vi "4. Panel Control.vi"   [LabVIEW 2017, in "1. Basic Panels.lvlib"]
uses:
  1. Basic Panels.lvlib
  panel-manager/Source/MGI-Panel Manager.lvlib
  panel-manager/Source/Panel/Subpanel/Subpanel.vi
  panel-manager/Source/Panel/Subpanel/Subpanel.lvclass
  panel-manager/Source/Panel/Window/Window.vi
  panel-manager/Source/Panel/Window/Window.lvclass
  panel-manager/Source/Window Position/Reference Position/Ref Top Level/Ref Top Level.vi
  panel-manager/Source/Window Position/Reference Position/Ref Top Level/Ref Top Level.lvclass
  panel-manager/Source/Window Position/Reference Position/Size/Absolute Size/Min Panel Size.vi
  panel-manager/Source/Window Position/Reference Position/Size/Absolute Size/Absolute Size.lvclass
  panel-manager/Source/Window Position/Reference Position/Alignment.ctl
  panel-manager/Source/Window Position/Reference Position/Reference Position.lvclass
  panel-manager/Source/Window Position/Reference Position/Offset/Absolute Offset/Absolute Offset.lvclass
  panel-manager/Source/Window Position/Reference Position/Vertical Alignment.ctl
  panel-manager/Source/Window Position/Reference Position/Horizontal Alignment.ctl
  D:/software/LabView_PanelManager/panel-manager/Source/Panel/Panel.lvclass
  D:/software/LabView_PanelManager/panel-manager/Source/Window Position/Reference Position/Offset/Offset.lvclass
  D:/software/LabView_PanelManager/panel-manager/Source/Window Position/Reference Position/Size/Size.lvclass
  D:/software/LabView_PanelManager/panel-manager/Source/Window Position/Reference Position/Reference Position.lvclass
  D:/software/LabView_PanelManager/panel-manager/Source/Window Position/Window Position.lvclass
panel:
  # "Run this VI to view instructions"
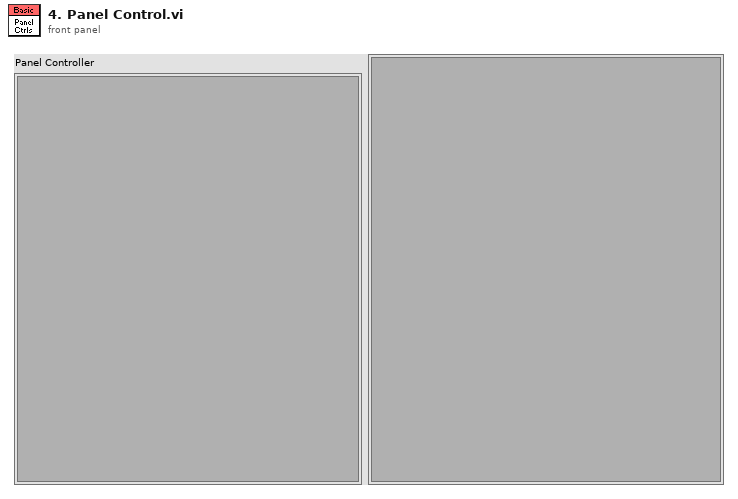
[diagram p1: front panel]
types:
  T1 = typedef "MGI-Panel Manager.lvlib/Reference Position.lvclass/Alignment.ctl" = cluster{"Horizontal":T2, "Vertical":T3}
  T2 = typedef "MGI-Panel Manager.lvlib/Reference Position.lvclass/Horizontal Alignment.ctl" = enum16{"Left", "Center", "Right"}
  T3 = typedef "MGI-Panel Manager.lvlib/Reference Position.lvclass/Vertical Alignment.ctl" = enum16{"Top", "Center", "Bottom"}
  T4 = typedef "LVRectTypeDef.ctl" = cluster{"Left":i16, "Top":i16, "Right":i16, "Bottom":i16}
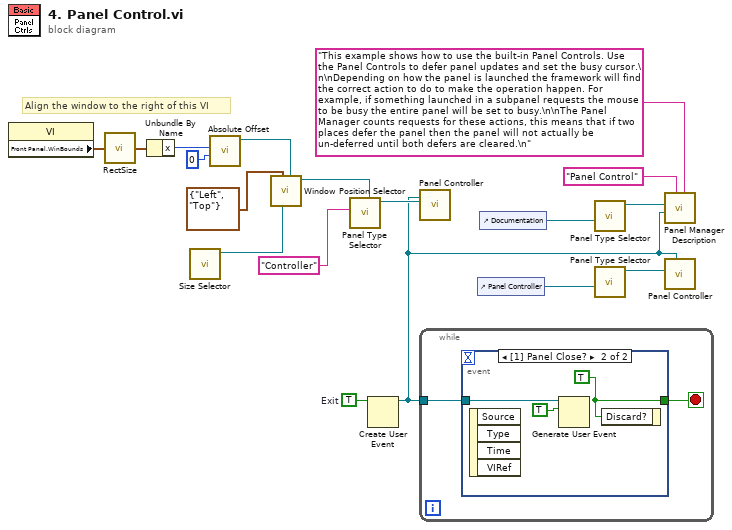
[diagram p0: block diagram]
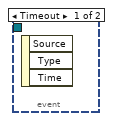
[diagram p2: hidden frame]
diagram:
  w16 = TRUE  # Exit
  # "Align the window to the right of this VI"
  n1 = property class="VI"() -> ("Front Panel.WinBounds"=w5:T4)  [unwired: 2 in, 2 out]
  n2 = call <vilib>:"RectSize.vi"("rect"=w5) -> ("point"=w4:cluster{"x":i16, "y":i16})
  n3 = Unbundle By Name(w4) -> ("x"=w3:i16)
  n4 = call-poly "Size Selector.vi"() -> ("Static out"=w8:refnum<class "Absolute Size.lvclass">)  [unwired: 10 in, 1 out]
  n5 = call "Absolute Offset.vi"("Vertical"=i16 0, "Horizontal"=w3) -> ("Absolute Offset Out"=w6:refnum<class "Absolute Offset.lvclass">)  [unwired: 8 in, 1 out]
  n6 = call-poly "Window Position Selector.vi"("Offset"=w6, "Size"=w8, "Alignment"=T1 {"Horizontal"=enum."Left", "Vertical"=enum."Top"}) -> ("Ref Top Level out"=w9:refnum<class "Ref Top Level.lvclass">)  [unwired: 7 in, 1 out]
  n7 = call-poly "Panel Type Selector.vi"("Window Position"=w9, "Default Title"="Controller") -> ("Window out"=w15:refnum<class "Window.lvclass">)  [unwired: 8 in, 1 out]
  n8 = Create User Event(user event datatype=w16) -> (user event=w11:refnum<user-event>)  [unwired: 1 in, 1 out]
  n9 = call "Panel Controller.vi"("Stop Event"=w11, "Panel"=w15) -> ()  [unwired: 10 in]
  n10 = while {
    tunnel: w11 -> [w19]
    stop <- w20 stop-if-true
    n11 = event shown="[1] Panel Close?" {
      selector: _ -> [_ _]
      dyn-events: _ -> [_ _]
      timeout: _ -> [_ _]
      tunnel: [_ w23] -> w20
      tunnel: w19 -> [_ w22]
      event Timeout {
        n12 = event-data() -> ()  [unwired: 1 in, 3 out]
      }
      event Panel Close? {
        w23 = TRUE ("Discard?")
        n13 = event-data() -> ()  [unwired: 1 in, 4 out]
        n14 = Generate User Event(user event=w22, event data cluster=TRUE ("event data")) -> ()  [unwired: 2 in, 2 out]
        n15 = event-data("Discard?"=w23) -> ()  [unwired: 1 in, 1 out]
      }
    }
  }
  n16 = control-ref of="Panel Controller"() -> (w18:refnum<vi>)
  n17 = control-ref of="Documentation"() -> (w13:refnum<vi>)
  n18 = call-poly "Panel Type Selector.vi"("Sub Panel"=w13) -> ("Subpanel Out"=w12:refnum<class "Subpanel.lvclass">)  [unwired: 9 in, 1 out]
  n19 = call-poly "Panel Type Selector.vi"("Sub Panel"=w18) -> ("Subpanel Out"=w17:refnum<class "Subpanel.lvclass">)  [unwired: 9 in, 1 out]
  n20 = call "Panel Manager Description.vi"("Description"="This example shows how to use the built-in Panel Controls. Use the Panel Controls to defer panel updates and set the busy cursor.\n\nDepending on how the panel is launched the framework will find the correct action to do to make the operation happen. For example, if something launched in a subpanel requests the mouse to be busy the entire panel will be set to busy.\n\nThe Panel Manager counts requests for these actions, this means that if two places defer the panel then the panel will not actually be un-deferred until both defers are cleared.\n" ("Description Title"), "Description Title"="Panel Control", "Stop Event"=w11, "Panel"=w12) -> ()  [unwired: 7 in, 1 out]
  n21 = call "Panel Controller.vi"("Stop Event"=w11, "Panel"=w17) -> ()  [unwired: 10 in]
